vi "handle message.vi"(8 "error in":errorcluster, 10 "message":refnum<class "communicator message.lvclass">, 11 "communicator in":refnum<class "communicator.lvclass">) -> (0 "error out":errorcluster, 1 "stop":bool, 3 "communicator out":refnum<class "communicator.lvclass">)   [LabVIEW 2015, in "communicator.lvclass"]
uses:
  communicator.lvclass
  message/communicator message.lvclass
  message/communicator message.lvclass/communicator message.ctl
  communicator.lvclass/communicator.ctl
  communicator queue/identifying queue.lvclass
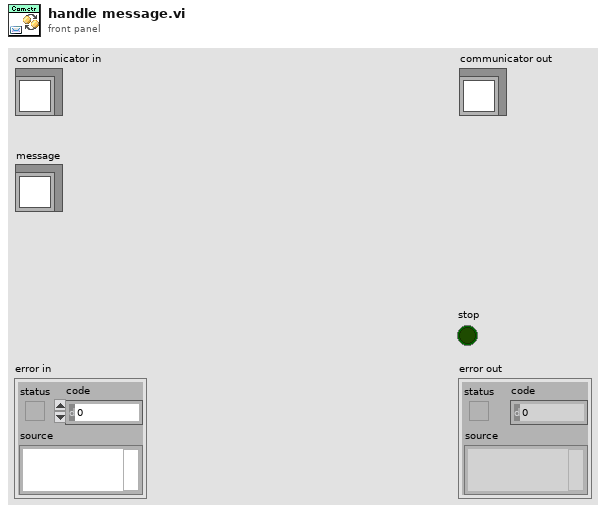
[diagram p1: front panel]
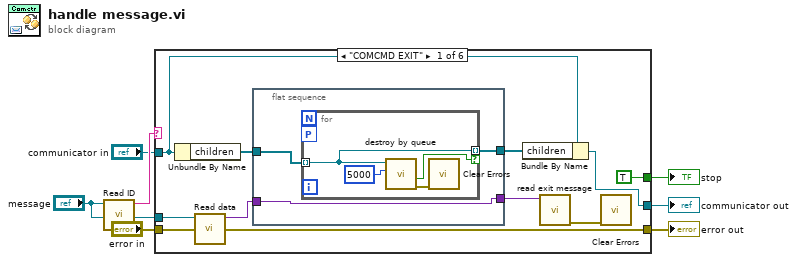
[diagram p0: block diagram]
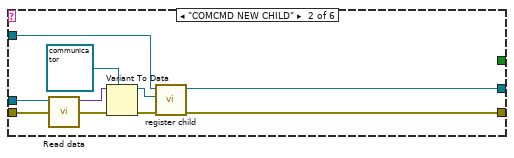
[diagram p2: hidden frame]
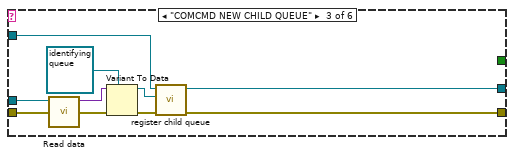
[diagram p3: hidden frame]
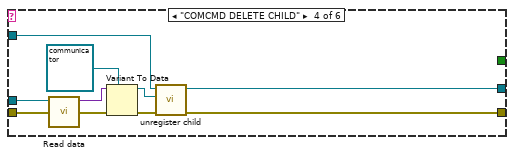
[diagram p4: hidden frame]
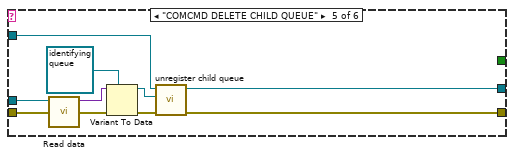
[diagram p5: hidden frame]
diagram:
  n1 = call "Read ID.vi"("communicator message in"="message") -> ("ID"=w7:string)  [unwired: 10 in]
  n2 = case shown="\"COMCMD EXIT\"" w7 {
    tunnel: "error in" -> [w15 w30 w39 w48 w57 w62]
    tunnel: [w15 w31 w40 w49 w58 w62] -> w5
    tunnel: "communicator in" -> [w13 w29 w38 w47 w56 w61]
    tunnel: [w9 w32 w41 w50 w59 w61] -> w3
    tunnel: "message" -> [w16 w33 w42 w51 w60 _]
    tunnel: [TRUE _ _ _ _ _] -> w1
    frame "COMCMD EXIT" {
      n3 = Unbundle By Name(w13) -> ("children"=w12:refnum<class "identifying queue.lvclass">[])
      n4 = call "Read data.vi"("communicator message in"=w16) -> ("data"=w10:variant)  [unwired: 10 in]
      n5 = flat-sequence {
        tunnel: w12 -> [w20]
        tunnel: [w19] -> w11
        tunnel: w10 -> [w19]
        tunnel: [w18] -> w8
        frame #0 {
          n6 = for {
            tunnel: w20 -> [w22] mode=indexing
            workers-P: _ -> [_]
            tunnel: [w22] -> w18 mode=indexing if=w21
            n7 = call "destroy by queue.vi"("timeout in ms (-1)"=5000, "queue"=w22) -> ("error out"=w23:errorcluster, "timed out?"=w21:bool)  [unwired: 8 in]
            n8 = call <vilib>:"Clear Errors.vi"("error in (no error)"=w23) -> ()  [unwired: 5 in, 2 out]
          }
        }
      }
      n9 = Bundle By Name(cluster=w13, "children"=w8) -> (w9:refnum<class "communicator.lvclass">)
      n10 = call "read exit message.vi"("data"=w11) -> ("error out"=w17:errorcluster)  [unwired: 10 in]
      n11 = call <vilib>:"Clear Errors.vi"("error in (no error)"=w17) -> ()  [unwired: 5 in, 2 out]
    }
    frame "COMCMD NEW CHILD" {
      n12 = call "Read data.vi"("communicator message in"=w33) -> ("data"=w27:variant)  [unwired: 10 in]
      n13 = Variant To Data(error in=w30, type=refnum<class "communicator.lvclass"> refnum ("communicator"), Variant=w27) -> (data=w26:refnum<class "communicator.lvclass">, error out=w28:errorcluster)
      n14 = call "register child.vi"("error in"=w28, "child"=w26, "communicator in"=w29) -> ("error out"=w31:errorcluster, "communicator out"=w32:refnum<class "communicator.lvclass">)  [unwired: 7 in]
    }
    frame "COMCMD NEW CHILD QUEUE" {
      n15 = call "Read data.vi"("communicator message in"=w42) -> ("data"=w36:variant)  [unwired: 10 in]
      n16 = Variant To Data(error in=w39, type=refnum<class "identifying queue.lvclass"> refnum ("identifying queue"), Variant=w36) -> (data=w34:refnum<class "identifying queue.lvclass">, error out=w37:errorcluster)
      n17 = call "register child queue.vi"("error in"=w37, "queue"=w34, "communicator in"=w38) -> ("error out"=w40:errorcluster, "communicator out"=w41:refnum<class "communicator.lvclass">)  [unwired: 7 in]
    }
    frame "COMCMD DELETE CHILD" {
      n18 = call "Read data.vi"("communicator message in"=w51) -> ("data"=w45:variant)  [unwired: 10 in]
      n19 = Variant To Data(error in=w48, type=refnum<class "communicator.lvclass"> refnum ("communicator"), Variant=w45) -> (data=w44:refnum<class "communicator.lvclass">, error out=w46:errorcluster)
      n20 = call "unregister child.vi"("error in"=w46, "child"=w44, "communicator in"=w47) -> ("error out"=w49:errorcluster, "communicator out"=w50:refnum<class "communicator.lvclass">)  [unwired: 7 in]
    }
    frame "COMCMD DELETE CHILD QUEUE" {
      n21 = call "Read data.vi"("communicator message in"=w60) -> ("data"=w54:variant)  [unwired: 10 in]
      n22 = Variant To Data(error in=w57, type=refnum<class "identifying queue.lvclass"> refnum ("identifying queue"), Variant=w54) -> (data=w52:refnum<class "identifying queue.lvclass">, error out=w55:errorcluster)
      n23 = call "unregister child queue.vi"("error in"=w55, "queue"=w52, "communicator in"=w56) -> ("error out"=w58:errorcluster, "communicator out"=w59:refnum<class "communicator.lvclass">)  [unwired: 7 in]
    }
    frame Default {
    }
  }
  "error out" <- w5
  "communicator out" <- w3
  "stop" <- w1
